vi "plot_main.vi"(10 "Break":refnum<vi>) -> ()   [LabVIEW 2019]
uses:
  controls/open_picButton.ctl
  controls/hydrolyse_picButton.ctl
  controls/methane_picButton.ctl
  controls/storage_picButton.ctl
  lib/libSimulationControl/libSimulationControl.lvlib
panel:
  in  "WindowTitle":string
  out "Load cluster":T1
  in  "Load Storage":T2 caption="Load Simulation"
  in  "Load Methane":T3 caption="Load Simulation"
  in  "Load Hydrolysis":T4 caption="Load Simulation"
  out "Output File Loaded?":bool
  in  "Close":bool
  out "# Lines Plot":i32
  in  "Parameters to Plot":string(tree)="_3"
  out "Output Files Path":path caption="selected path"
  in  "Load File":T5
  in  "Clear Plot Selection":bool
  in  "Plot":bool
  # "Biogas Plotter"
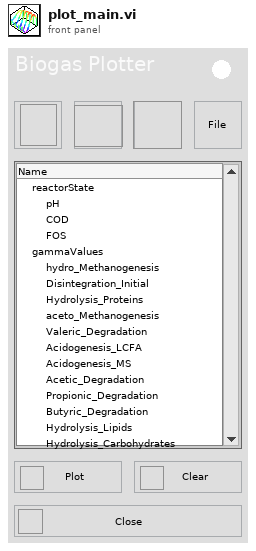
[diagram p1: front panel]
types:
  T1 = cluster{"# Lines Plot":refnum<vi>, "Output File Loaded?":refnum<vi>, "Parameters to Plot":refnum<vi>, "Output Files Path":refnum<vi>}
  T2 = typedef "storage_picButton.ctl" = bool
  T3 = typedef "methane_picButton.ctl" = bool
  T4 = typedef "hydrolyse_picButton.ctl" = bool
  T5 = typedef "open_picButton.ctl" = bool
  T6 = typedef "LVPoint32TypeDef.ctl" = cluster{"Horizontal":i32, "Vertical":i32}
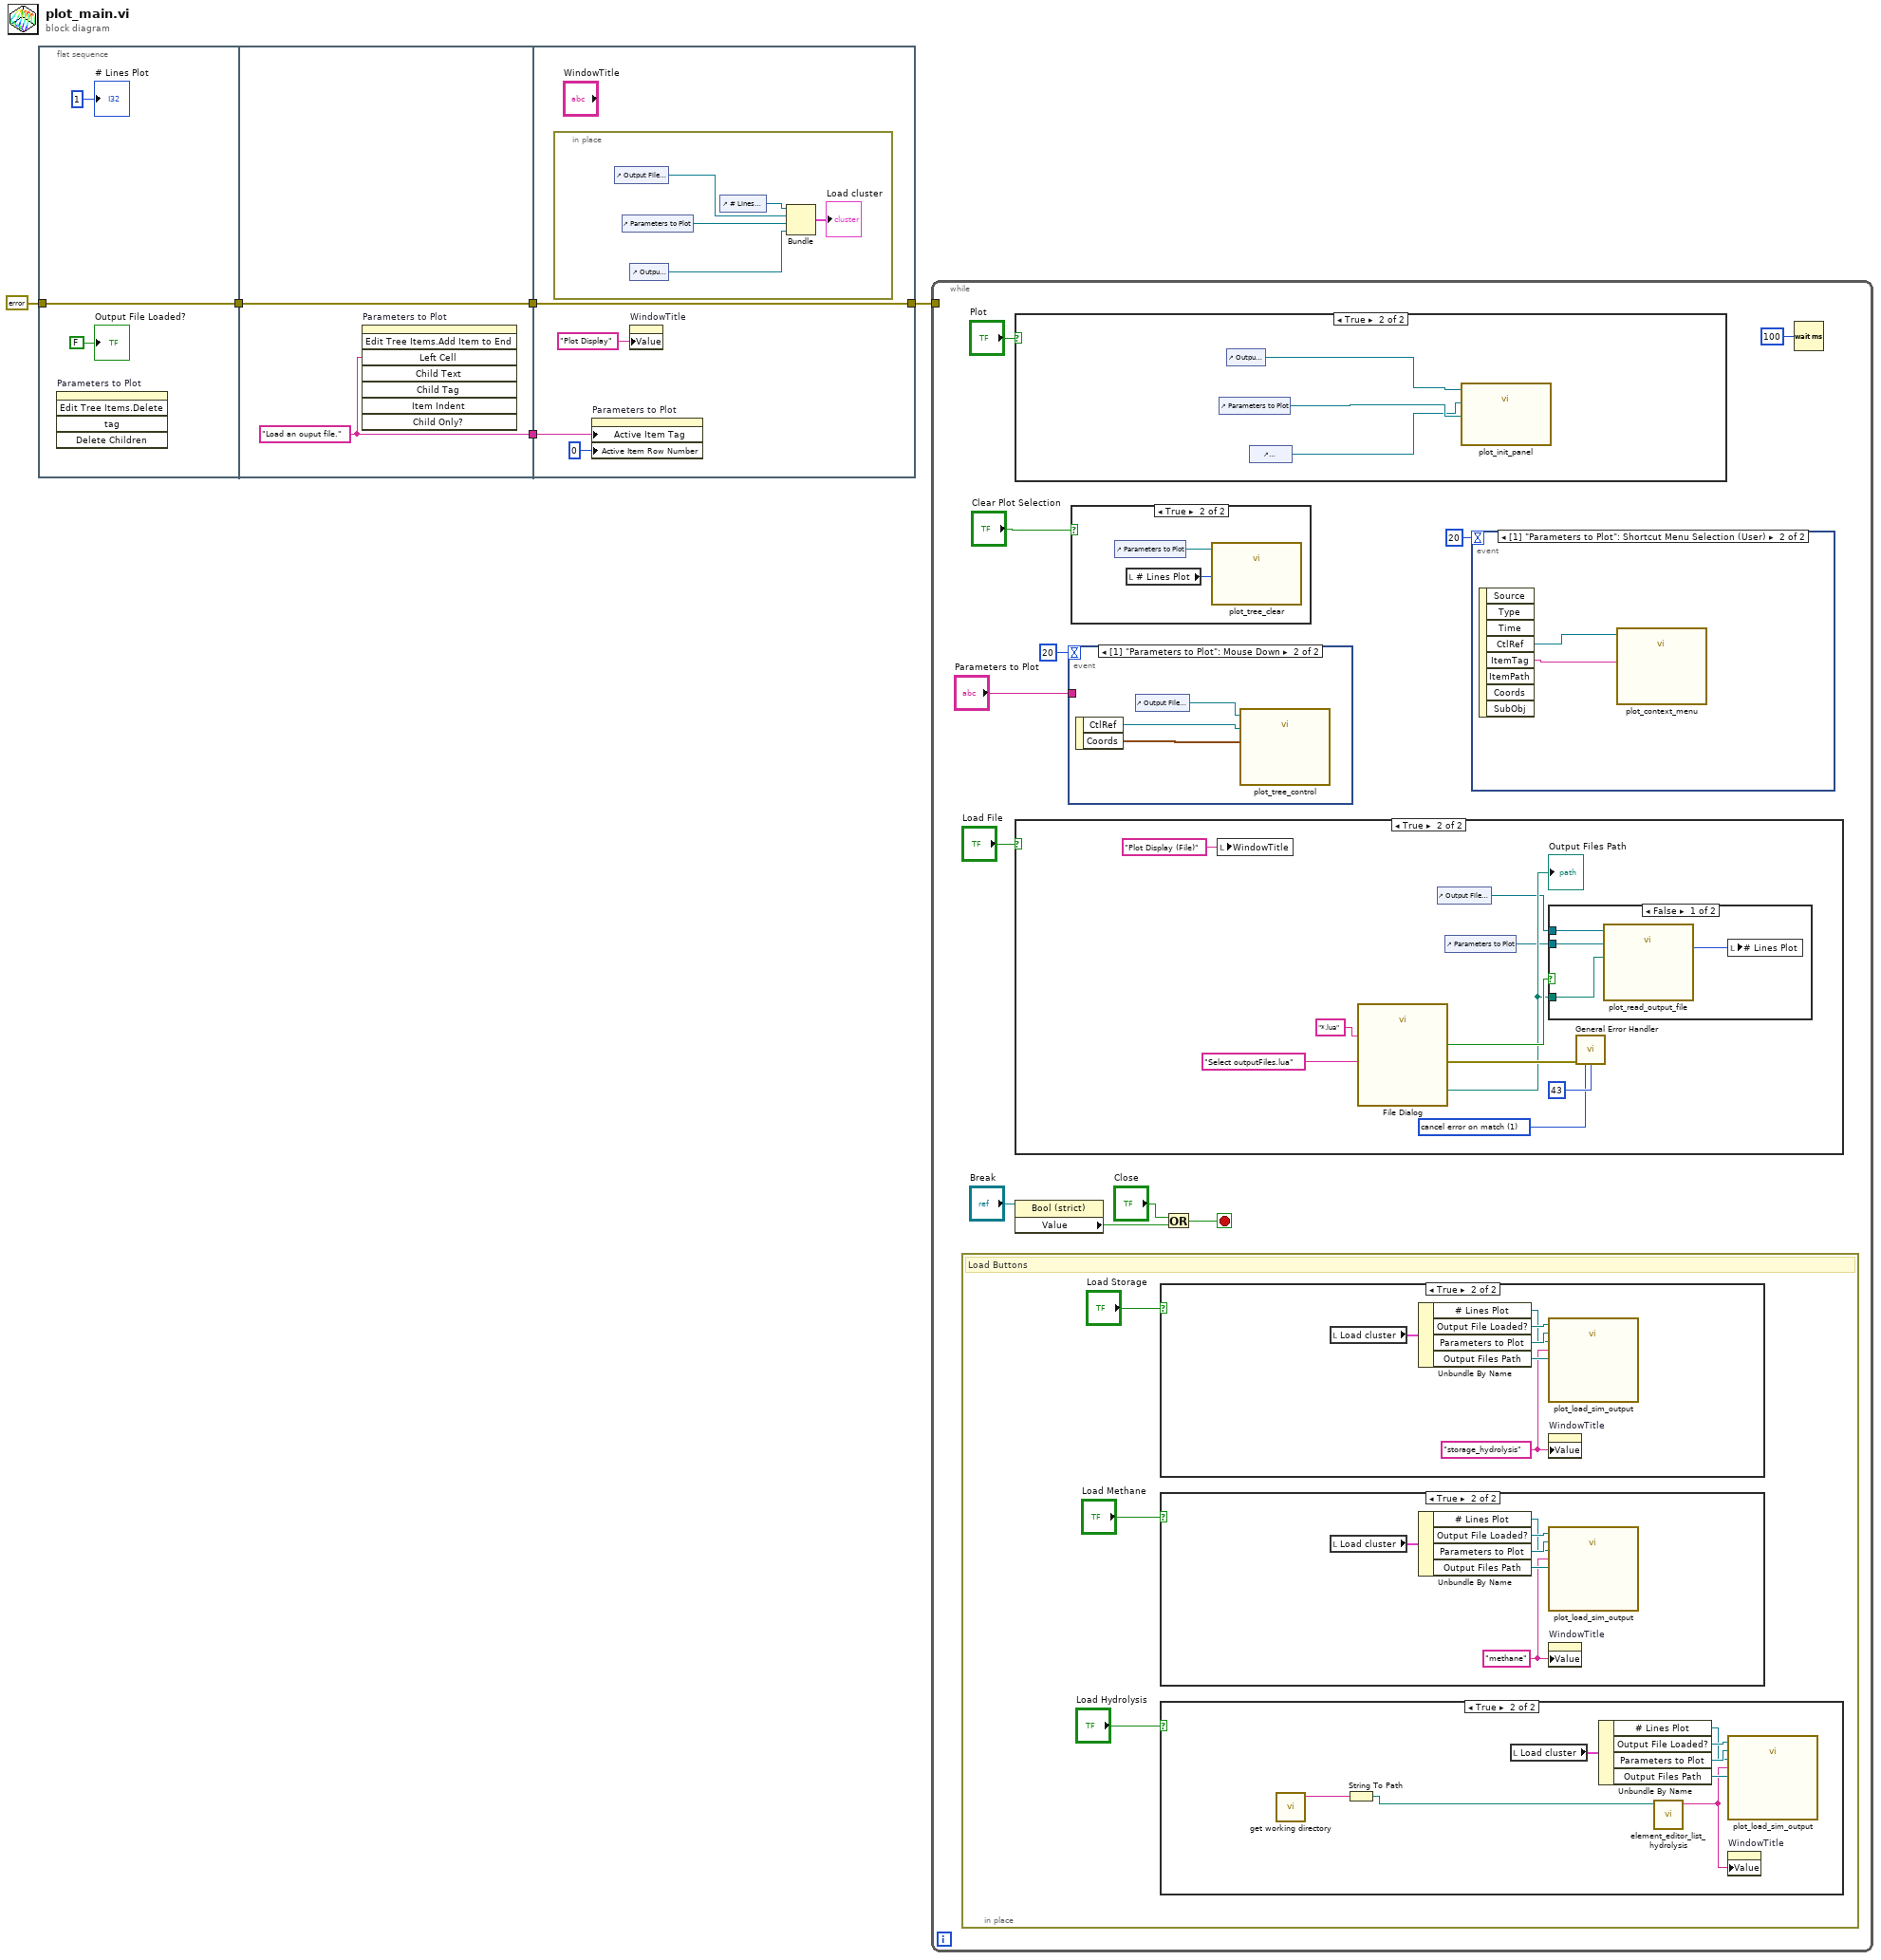
[diagram p0: block diagram]
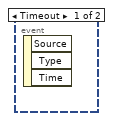
[diagram p2: hidden frame]
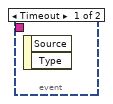
[diagram p9: hidden frame]
diagram:
  n1 = flat-sequence {
    tunnel: [w6] -> w3
    tunnel: errorcluster {"status"=FALSE, "code"=0, "source"=""} ("error constant") -> [w6]
    tunnel: [w10] -> w5
    tunnel: w3 -> [w9]
    tunnel: [w9] -> w2
    tunnel: w5 -> [w14]
    tunnel: w2 -> [w12]
    tunnel: [w12] -> w1
    frame #0 {
      n2 = invoke on="Parameters to Plot" class="Tree (strict)" method="Edit Tree Items.Delete"() -> ()  [unwired: 5 in, 5 out]
      "Output File Loaded?" <- FALSE ("Output File Loaded?")
      "# Lines Plot" <- 1 ("# Lines Plot")
    }
    frame #1 {
      w10 = "Load an ouput file." ("Left Cell String")
      n3 = invoke on="Parameters to Plot" class="Tree (strict)" method="Edit Tree Items.Add Item to End"("Left Cell"=w10) -> ()  [unwired: 7 in, 8 out]
    }
    frame #2 {
      n4 = in-place {
        n5 = control-ref of="Output File Loaded?"() -> (w18:refnum<vi>)
        n6 = control-ref of="Parameters to Plot"() -> (w17:refnum<vi>)
        n7 = control-ref of="Output Files Path"() -> (w16:refnum<vi>)
        n8 = control-ref of="# Lines Plot"() -> (w19:refnum<vi>)
        n9 = Bundle("# Lines Plot"=w19, "Output File Loaded?"=w18, "Parameters to Plot"=w17, "Output Files Path"=w16) -> (→"Load cluster":T1)  [unwired: 1 in]
      }
      n10 = property on="Parameters to Plot" class="Tree (strict)"("Active Item Tag"=w14, "Active Item Row Number"=0 ("Active Item:Row Number")) -> ()  [unwired: 2 in, 2 out]
      n11 = property on="WindowTitle" class="Str"("Value"="Plot Display" ("WindowTitle")) -> ()  [unwired: 2 in, 2 out]
    }
  }
  n12 = while {
    tunnel: w1 -> [_]
    stop <- w22 stop-if-true
    n13 = in-place {
      # "Load Buttons"
      n14 = case shown="True" "Load Storage" {
        frame False {
        }
        frame True {
          w36 = "storage_hydrolysis" ("Folder")
          n15 = local read "Load cluster"() -> (w41:T1)
          n16 = Unbundle By Name(w41) -> ("# Lines Plot"=w38:refnum<vi>, "Output File Loaded?"=w40:refnum<vi>, "Parameters to Plot"=w39:refnum<vi>, "Output Files Path"=w37:refnum<vi>)
          n17 = call "plot_load_sim_output.vi"("Output Files Path"=w37, "Folder"=w36, "# Lines Plot"=w38, "Parameters to Plot"=w39, "Output File Loaded?"=w40) -> ()  [unwired: 7 in]
          n18 = property on="WindowTitle" class="Str"("Value"=w36) -> ()  [unwired: 2 in, 2 out]
        }
      }
      n19 = case shown="True" "Load Methane" {
        frame False {
        }
        frame True {
          w50 = "methane" ("Folder")
          n20 = local read "Load cluster"() -> (w55:T1)
          n21 = Unbundle By Name(w55) -> ("# Lines Plot"=w52:refnum<vi>, "Output File Loaded?"=w54:refnum<vi>, "Parameters to Plot"=w53:refnum<vi>, "Output Files Path"=w51:refnum<vi>)
          n22 = call "plot_load_sim_output.vi"("Output Files Path"=w51, "Folder"=w50, "# Lines Plot"=w52, "Parameters to Plot"=w53, "Output File Loaded?"=w54) -> ()  [unwired: 7 in]
          n23 = property on="WindowTitle" class="Str"("Value"=w50) -> ()  [unwired: 2 in, 2 out]
        }
      }
      n24 = case shown="True" "Load Hydrolysis" {
        frame False {
        }
        frame True {
          n25 = call "get working directory.vi"() -> ("function return"=w44:string)  [unwired: 10 in, 1 out]
          n26 = String To Path(string=w44) -> (path=w42:path)
          n27 = local read "Load cluster"() -> (w49:T1)
          n28 = Unbundle By Name(w49) -> ("# Lines Plot"=w46:refnum<vi>, "Output File Loaded?"=w48:refnum<vi>, "Parameters to Plot"=w47:refnum<vi>, "Output Files Path"=w45:refnum<vi>)
          n29 = call "element_editor_list_hydrolysis.vi"("path"=w42) -> ("Value"=w43:string)  [unwired: 7 in, 3 out]
          n30 = call "plot_load_sim_output.vi"("Output Files Path"=w45, "Folder"=w43, "# Lines Plot"=w46, "Parameters to Plot"=w47, "Output File Loaded?"=w48) -> ()  [unwired: 7 in]
          n31 = property on="WindowTitle" class="Str"("Value"=w43) -> ()  [unwired: 2 in, 2 out]
        }
      }
    }
    n32 = case shown="True" "Plot" {
      frame False {
      }
      frame True {
        n33 = control-ref of="Parameters to Plot"() -> (w57:refnum<vi>)
        n34 = control-ref of="Output Files Path"() -> (w58:refnum<vi>)
        n35 = control-ref of="WindowTitle"() -> (w56:refnum<vi>)
        n36 = call "plot_init_panel.vi"("Plot Tree"=w57, "Window Title"=w56, "Output Files Path"=w58) -> ()  [unwired: 9 in]
      }
    }
    n37 = case shown="True" "Load File" {
      frame False {
      }
      frame True {
        w66 = 1 items=["no exception", "cancel error on match", "set error on match"] ("[exception action] (none:0)")
        n38 = local write "WindowTitle"("Plot Display (File)" ("WindowTitle")) -> ()
        n39 = call "File Dialog"("prompt"="Select outputFiles.lua", "pattern (all files)"="*.lua") -> ("selected path"=w64:path, "cancelled"=w65:bool, "error out"=w68:errorcluster)  [unwired: 10 in, 1 out]
        "Output Files Path" <- w64
        n40 = control-ref of="Output File Loaded?"() -> (w62:refnum<vi>)
        n41 = control-ref of="Parameters to Plot"() -> (w63:refnum<vi>)
        n42 = case shown="False" w65 {
          tunnel: w64 -> [w72 _]
          tunnel: w63 -> [w71 _]
          tunnel: w62 -> [w70 _]
          frame False {
            n43 = call "plot_read_output_file.vi"("TMP Filepath"=w72, "Plot Tree"=w71, "Output File Loaded?"=w70) -> ("# Lines Plot"=w69:i32)  [unwired: 8 in]
            n44 = local write "# Lines Plot"(w69) -> ()
          }
          frame True {
          }
        }
        n45 = call <vilib>:"General Error Handler.vi"("error in (no error)"=w68, "[exception action] (none:0)"=w66, "[exception code]"=43) -> ()  [unwired: 8 in, 5 out]
      }
    }
    n46 = property class="Bool (strict)"(reference="Break") -> ("Value"=w23:bool)  [unwired: 1 in, 2 out]
    n47 = event shown="[1] \"Parameters to Plot\": Mouse Down" {
      selector: _ -> [_ _]
      dyn-events: _ -> [_ _]
      timeout: 20 -> [_ _]
      tunnel: "Parameters to Plot" -> [_ _]
      event Timeout {
        n48 = event-data() -> ()  [unwired: 1 in, 2 out]
      }
      event "Parameters to Plot": Mouse Down {
        n49 = event-data() -> ("CtlRef"=w75:refnum<vi>, "Coords"=w74:T6)  [unwired: 1 in]
        n50 = control-ref of="Output File Loaded?"() -> (w73:refnum<vi>)
        n51 = call "plot_tree_control.vi"("Point"=w74, "Plot Tree"=w75, "Output File Loaded?"=w73) -> ()  [unwired: 9 in]
      }
    }
    n52 = case shown="True" "Clear Plot Selection" {
      frame False {
      }
      frame True {
        n53 = control-ref of="Parameters to Plot"() -> (w76:refnum<vi>)
        n54 = local read "# Lines Plot"() -> (w77:i32)
        n55 = call "plot_tree_clear.vi"("# Lines Plot"=w77, "Plot Tree"=w76) -> ()  [unwired: 10 in]
      }
    }
    n56 = Or(x="Close", y=w23) -> (x .or. y?=w22:bool)
    n57 = event shown="[1] \"Parameters to Plot\": Shortcut Menu Selection (User)" {
      selector: _ -> [_ _]
      dyn-events: _ -> [_ _]
      timeout: 20 -> [_ _]
      event Timeout {
        n58 = event-data() -> ()  [unwired: 1 in, 3 out]
      }
      event "Parameters to Plot": Shortcut Menu Selection (User) {
        n59 = event-data() -> ("CtlRef"=w31:refnum<vi>, "ItemTag"=w32:string)  [unwired: 1 in, 6 out]
        n60 = call "plot_context_menu.vi"("MenuSelection"=w32, "Tree"=w31) -> ()  [unwired: 10 in]
      }
    }
    n61 = Wait (ms)(milliseconds to wait=u32 100) -> ()  [unwired: 1 out]
  }
